vi "FGV_ToProductionScreenEvent.vi"(7 "Command":T1, 8 "error in":errorcluster) -> (0 "error out":errorcluster, 3 "ToProductionScreenEvent":refnum<user-event>)   [LabVIEW 2011]
uses:
  EnumFgvEventCommand.ctl
  ToProductionScreenEvent.ctl
  ToProductionScreenEvent_Orders.ctl
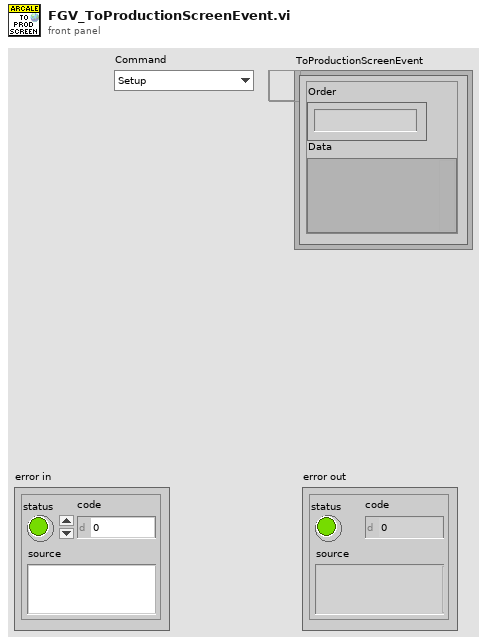
[diagram p1: front panel]
types:
  T1 = typedef "EnumFgvEventCommand.ctl" = enum16{"Setup", "Cleanup", "Get"}
  T2 = typedef "ToProductionScreenEvent.ctl" = cluster{"Order":T3, "Data":variant}
  T3 = typedef "ToProductionScreenEvent_Orders.ctl" = enum16{"Progress Percentage Update", "NaO", "Get PreUUT Notifier Ref", "PM execution over", "Update list of Tests", "Test Name And Result", "Test UUT Progress", "Global Test Result and Exec Time", "Scripting Starts", "Scripting Ends", "UUT Test Starts", "DB Log Starts", "DB Log Ends", "MES UUT Check Starts", "MES UUT Check Ends", "MES UUT Status Starts", "MES UUT Status Ends", "MES UUT Results Starts", "MES UUT Results Ends", "Opening Inst Ref", "End Opening Inst Ref", "Update Spec Name"}
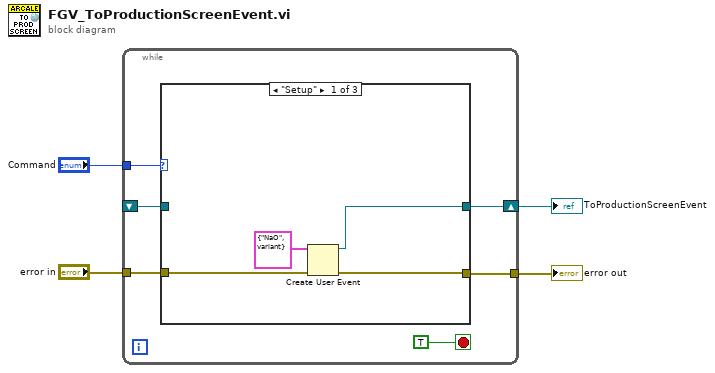
[diagram p0: block diagram]
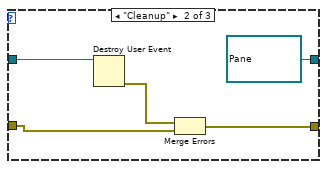
[diagram p2: hidden frame]
diagram:
  n1 = while {
    tunnel: "error in" -> [w8]
    tunnel: "Command" -> [w9]
    tunnel: [w7] -> w2
    shift-right: [w6] -> w1
    shift-left: _ -> [w5]
    stop <- TRUE stop-if-true
    n2 = case shown="\"Setup\"" w9 {
      tunnel: w8 -> [w14 w18 w20]
      tunnel: [w13 w16 w20] -> w7
      tunnel: [w12 refnum<user-event> refnum ("ToProductionScreenEvent") w21] -> w6
      tunnel: w5 -> [_ w19 w21]
      frame "Setup" {
        n3 = Create User Event(user event datatype=T2 {"Order"=enum."NaO", "Data"=variant} ("ToProductionScreenEvent"), error in=w14) -> (user event=w12:refnum<user-event>, error out=w13:errorcluster)
      }
      frame "Cleanup" {
        n4 = Destroy User Event(user event=w19) -> (error out=w17:errorcluster)  [unwired: 1 in]
        n5 = Merge Errors(w17, w18) -> (w16:errorcluster)
      }
      frame "Get" {
      }
    }
  }
  "error out" <- w2
  "ToProductionScreenEvent" <- w1
